vi "Queue_Close.vi"(8 "Error In":errorcluster, 11 "Response Queue":refnum<queue>) -> (0 "Error Out":errorcluster)   [LabVIEW 2018, in "HttpClient_NET.lvlib" / "HttpClient_NET.lvclass"]
doc: "<b> </b> <b> </b>\nHttpClient_NET\nJustin Young - Viviota\nCopyright (c) 2021\nLicense: BSD"
uses:
  HttpClient_NET.lvclass
  HttpResponseMessage/Types/ResponseMessage_Cluster.ctl
  HttpResponseMessage/HttpResponseMessage.lvclass
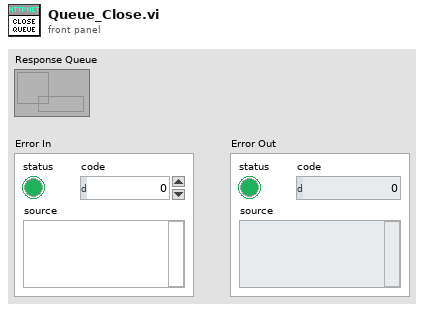
[diagram p1: front panel]
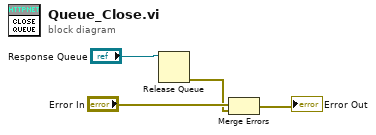
[diagram p0: block diagram]
diagram:
  n1 = Release Queue(queue="Response Queue") -> (error out=w1:errorcluster)  [unwired: 2 in, 2 out]
  n2 = Merge Errors("Error In", w1) -> (→"Error Out":errorcluster)
